vi "Write to File.vi"(7 "Direction":string, 8 "error in (no error)":errorcluster, 10 "Channels":refnum<class "Channel.lvclass">[](array[class]), 11 "TXT in":refnum<class "TXT.lvclass">) -> (0 "error out":errorcluster, 3 "TXT out":refnum<class "TXT.lvclass">)   [LabVIEW 2020, in "TXT.lvlib" / "TXT.lvclass"]
uses:
  TXT.lvclass
  built/windows/Channel.lvlibp/Channel.lvclass
  TXT.lvclass/TXT.ctl
  TXT Global.vi
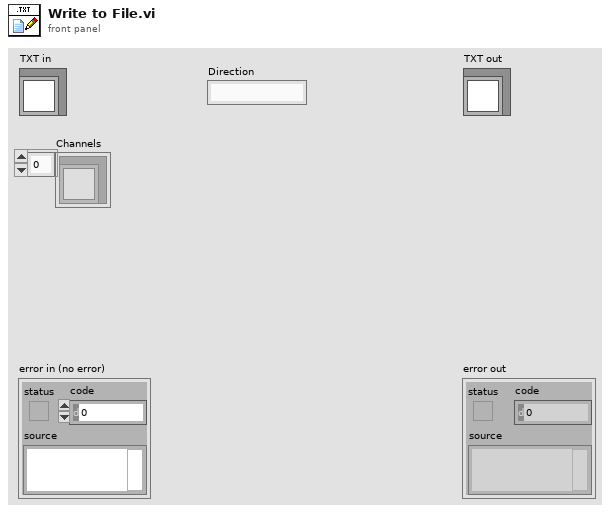
[diagram p1: front panel]
types:
  T1 = typedef "Channel.lvlibp/NI_Data Type.lvlib/Data Type.ctl" = enum8{"Invalid Type", "Void", "I8", "I16", "I32", "I64", "U8", "U16", "U32", "U64", "Single Float", "Double Float", "Extended Float", "Single Complex", "Double Complex", "Extended Complex", "Enum U8", "Enum U16", "Enum U32", "Enum U64", "Single Float With Unit", "Double Float With Unit", "Extended Float With Unit", "Single Complex with Unit", "Double Complex with Unit", "Extended Complex with Unit", "Boolean", "String", "Path", "Picture", "Tag", "Array", "Cluster", "Variant", "LV Variant", "Waveform", "Timestamp", "Digital Waveform", "Digital Data", "ExpressData", "Refnum", "External Data", "VI", "Poly VI", "LabVIEW Class Instance", "Fixed Point", "Set Collection", "Map Collection"}
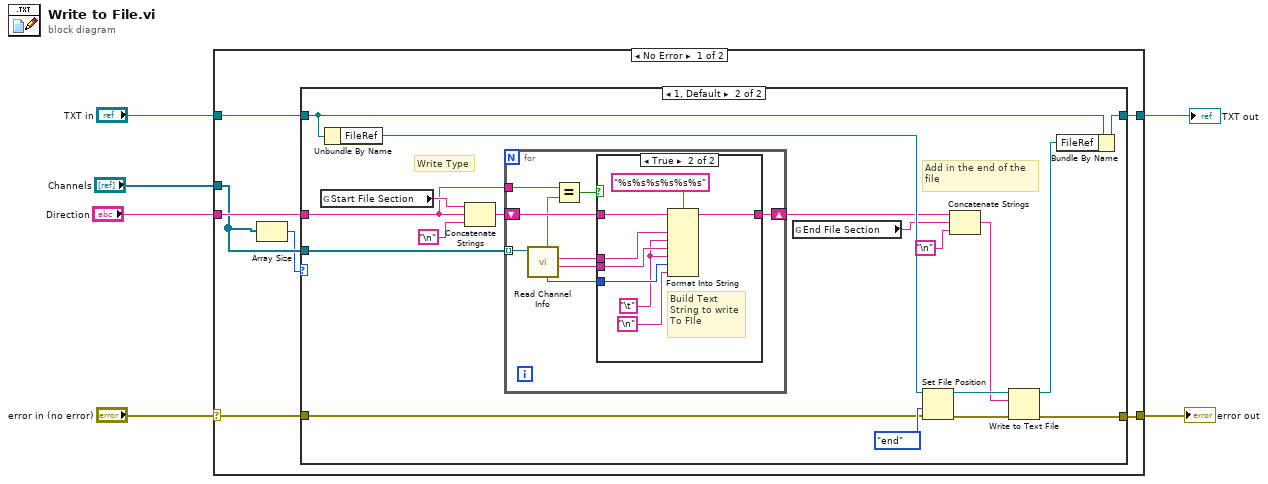
[diagram p0: block diagram]
diagram:
  n1 = case shown="No Error" "error in (no error)" {
    selector: "error in (no error)" -> [w10 w53]
    tunnel: [w12 w53] -> w5
    tunnel: "TXT in" -> [w13 w52]
    tunnel: [w11 w52] -> w3
    tunnel: "Channels" -> [w8 _]
    tunnel: "Direction" -> [w9 _]
    frame No Error {
      n2 = Array Size(array=w8) -> (size(s)=w7:i32)
      n3 = case shown="1, Default" w7 {
        tunnel: w13 -> [w15 w33]
        tunnel: [w14 w31] -> w12
        tunnel: [w15 w26] -> w11
        tunnel: w10 -> [w14 w18]
        tunnel: w9 -> [_ w17]
        tunnel: w8 -> [_ w16]
        frame 0 {
        }
        frame 1, Default {
          # "Add in the end of the\nfile"
          # "Write Type"
          n4 = global read "TXT Global.vi" "Start File Section"() -> (w23:string)
          n5 = Unbundle By Name(w33) -> ("FileRef"=w29:refnum<file>)
          n6 = Concatenate Strings(w23, w17, "\n") -> (w24:string)
          n7 = for {
            tunnel: w16 -> [w42] mode=indexing
            shift-right: [w40] -> w22
            shift-left: w24 -> [w41]
            tunnel: w17 -> [w36]
            n8 = call "Read Channel Info.vi"("Channel in"=w42) -> ("URL"=w38:string, "Name"=w39:string, "DataType"=w37:T1, "Read or Write"=w35:string)  [unwired: 5 in, 2 out]
            n9 = Equal?(x=w36, y=w35) -> (x = y?=w34:bool)
            n10 = case shown="True" w34 {
              tunnel: w41 -> [w43 w51]
              tunnel: [w43 w50] -> w40
              tunnel: w39 -> [_ w49]
              tunnel: w38 -> [_ w48]
              tunnel: w37 -> [_ w47]
              frame False {
              }
              frame True {
                w46 = "\t"
                # "Build Text\nString to write\nTo FIle"
                n11 = Format Into String(format string="%s%s%s%s%s%s", initial string=w51, w49, w46, w48, w46, w47, "\n") -> (resulting string=w50:string)  [unwired: 1 in, 1 out]
              }
            }
          }
          n12 = global read "TXT Global.vi" "End File Section"() -> (w19:string)
          n13 = Set File Position(refnum=w29, from (0:start)=enum16{"start", "end", "current"}."end", error in=w18) -> (refnum out=w28:refnum<file>, error out=w27:errorcluster)  [unwired: 1 in]
          n14 = Concatenate Strings(w22, w19, "\n") -> (w21:string)
          n15 = Write to Text File(file (use dialog)=w28, text=w21, error in=w27) -> (refnum out=w25:refnum<file>, error out=w31:errorcluster)  [unwired: 1 in, 1 out]
          n16 = Bundle By Name(cluster=w33, "FileRef"=w25) -> (w26:refnum<class "TXT.lvclass">)
        }
      }
    }
    frame Error {
    }
  }
  "error out" <- w5
  "TXT out" <- w3
